vi "Input File Run or Stop.vi"(7 "timeout":i32=200, 8 "error in (no error)":errorcluster, 11 "MM Button Events In":refnum<notifier>) -> (0 "error out":errorcluster, 1 "Running":T1=enum."Run", 3 "Button Events Out":refnum<notifier>)   [LabVIEW 2009]
uses:
  MixedMode/Messages/Mixed Mode Button Events Message.ctl
  MixedMode/Messages/Mixed Mode Button Events.ctl
  Mixed Mode Widget Button States.ctl
  Run Or Stop Result.ctl
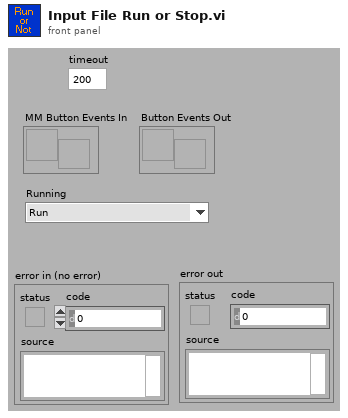
[diagram p1: front panel]
types:
  T1 = typedef "Run Or Stop Result.ctl" = enum16{"Nevermind", "Run", "Stop"}
  T2 = typedef "Mixed Mode Button Events Message.ctl" = cluster{"MM Control Events":T3, "Button States":T4}
  T3 = typedef "Mixed Mode Button Events.ctl" = enum16{"Propose.Accept", "Propose.Decline", "Execute.Start", "Execute.Stop", "TargetSet", "InputFile.Load", "InputFile.Reset", "InputFile.Pause", "InputFile.Run", "CartesianType.Changed", "NCTP.ConnectToServer", "NTCP.DisconnectFromServer", "Application.Stop", "Control.Enabled", "Control.Disabled", "ControlType.Changed", "Nop"}
  T4 = typedef "Mixed Mode Widget Button States.ctl" = cluster{"Auto-Start Enabled":bool, "Auto-Accept Enabled":bool, "Exit Requested":bool, "Input File Loaded":bool, "Input File Running":bool, "NTCP Server  On":bool}
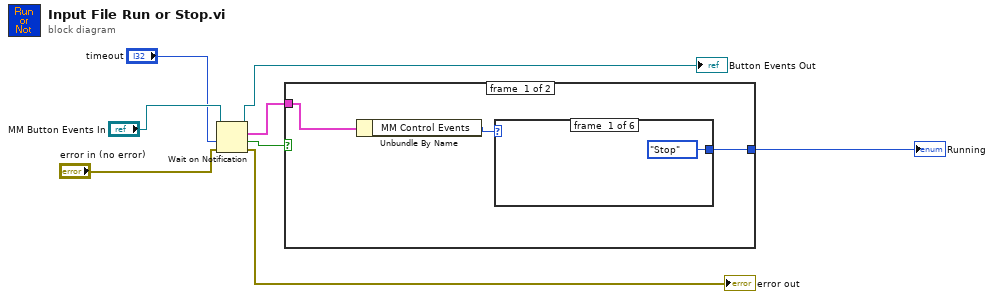
[diagram p0: block diagram]
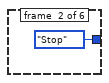
[diagram p2: hidden frame]
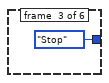
[diagram p3: hidden frame]
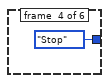
[diagram p4: hidden frame]
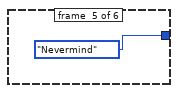
[diagram p5: hidden frame]
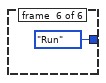
[diagram p6: hidden frame]
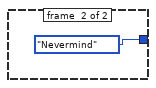
[diagram p7: hidden frame]
diagram:
  n1 = Wait on Notification(notifier="MM Button Events In", timeout in ms (-1)="timeout", error in (no error)="error in (no error)") -> (notifier out=→"Button Events Out":refnum<notifier>, notification=w3:T2, timed out?=w4:bool, error out=→"error out":errorcluster)  [unwired: 1 in]
  n2 = case shown="False" w4 {
    tunnel: w3 -> [w11 _]
    tunnel: [w9 Run_Or_Stop_Result."Nevermind" ("Running")] -> w1
    frame #0 {
      n3 = Unbundle By Name(w11) -> ("MM Control Events"=w10:T3)
      n4 = case shown="\"Nop\", Default" w10 {
        tunnel: [Run_Or_Stop_Result."Stop" ("Running") Run_Or_Stop_Result."Stop" ("Running") Run_Or_Stop_Result."Stop" ("Running") Run_Or_Stop_Result."Stop" ("Running") Run_Or_Stop_Result."Nevermind" ("Running") Run_Or_Stop_Result."Run" ("Running")] -> w9
        frame #0 {
        }
        frame #1 {
        }
        frame #2 {
        }
        frame #3 {
        }
        frame #4 {
        }
        frame #5 {
        }
      }
    }
    frame #1 {
    }
  }
  "Running" <- w1
